vi "Apply Protection.vi"(8 "error in":errorcluster, 11 "6032A in":refnum<class "6032A.lvclass">) -> (0 "error out":errorcluster, 3 "6032A out":refnum<class "6032A.lvclass">)   [LabVIEW 2019, in "6032A.lvlib" / "6032A.lvclass"]
uses:
  Library/6032A.lvclass
  C:/Users/Public/Documents/Development/builds/Instruments/PowerSupply.lvlibp/Library/PowerSupply.lvclass
  Library/6032A.lvclass/6032A.ctl
  <instrlib>/Agilent 6XXX Series/Agilent 6XXX Series.lvlib
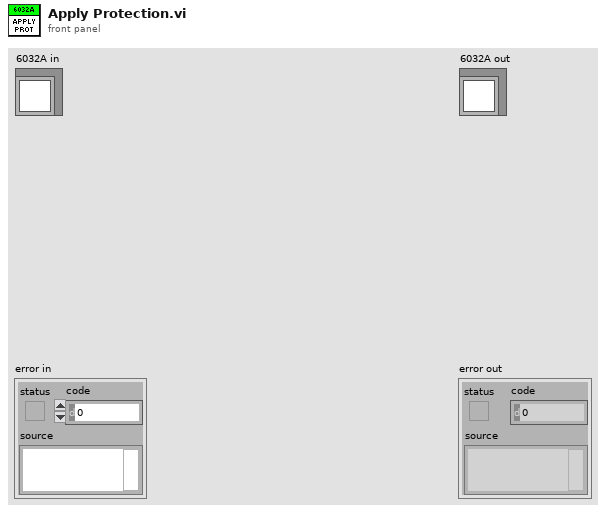
[diagram p1: front panel]
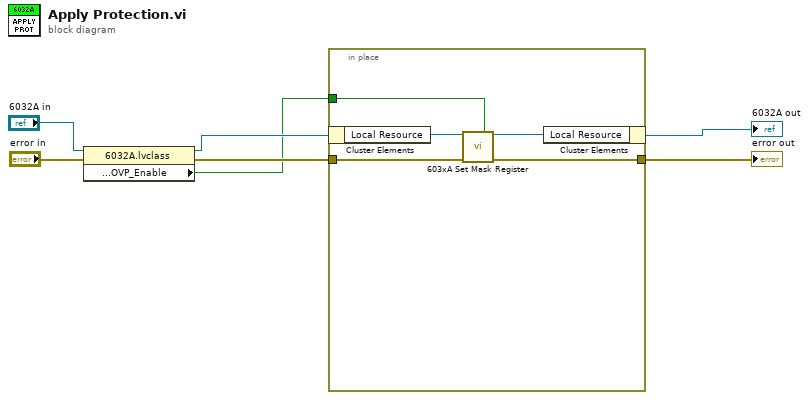
[diagram p0: block diagram]
diagram:
  n1 = property class="6032A.lvclass"(reference="6032A in", error in="error in") -> (reference out=w4:refnum<class "6032A.lvclass">, error out=w3:errorcluster, "Accessors:Setting:Protection:OVP_Enable"=w1:bool)
  n2 = in-place {
    in-place-border: [w10] -> w6
    in-place-border: w3 -> [w9]
    in-place-border: w1 -> [w8]
    n3 = in-place-cluster #1(w4) -> ("Local Resource"=w12:refnum<visa-resource-name>)
    n4 = call <instrlib>:"603xA Set Mask Register.vi"("VISA resource name"=w12, "overvoltage (F:off)"=w8, "error in (no error)"=w9) -> ("VISA resource name out"=w11:refnum<visa-resource-name>, "error out"=w10:errorcluster)  [unwired: 11 in]
    n5 = in-place-cluster #1("Local Resource"=w11) -> (→"6032A out":refnum<class "6032A.lvclass">)
  }
  "error out" <- w6
